vi "Bar graph with LEDs.vi"() -> ()   [LabVIEW 2010]
doc: "This example shows how to make a bar graph by controlling Red Pitaya on board LEDs.\nThe number of LEDs that will be turned ON, corresponds to the value of variable p."
uses:
  RedPitaya.lvlib
panel:
  in  "stop":bool
  in  "Percent":i32 min=0 max=100
  in  "IP address":string="192.168.4.129"
  # "Enter a value between 0 and 100%"
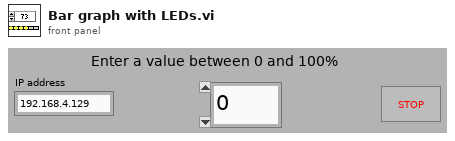
[diagram p1: front panel]
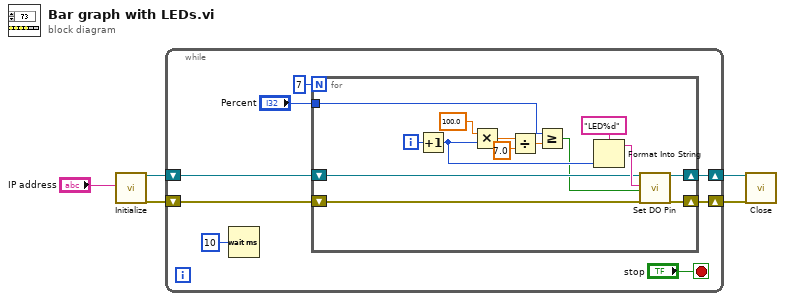
[diagram p0: block diagram]
diagram:
  n1 = call "Initialize.vi"("IP address"="IP address") -> ("RedPitaya connection out"=w2:refnum<k5>, "error out"=w1:errorcluster)  [unwired: 17 in]
  n2 = while {
    shift-right: [w12] -> w4
    shift-left: w2 -> [w10]
    shift-right: [w11] -> w3
    shift-left: w1 -> [w9]
    stop <- "stop" stop-if-true
    n3 = Wait (ms)(milliseconds to wait=u32 10) -> ()  [unwired: 1 out]
    n4 = for {
      N: 7 -> [_]
      tunnel: "Percent" -> [w23]
      shift-right: [w17] -> w12
      shift-left: w10 -> [w18]
      shift-right: [w16] -> w11
      shift-left: w9 -> [w19]
      i -> [w21]
      n5 = Increment(x=w21) -> (x+1=w15:i32)
      n6 = Multiply(x=100.0, y=w15) -> (x*y=w25:dbl)
      n7 = Divide(x=w25, y=7.0) -> (x/y=w27:dbl)
      n8 = Greater Or Equal?(x=w23, y=w27) -> (x >= y?=w14:bool)
      n9 = Format Into String(format string="LED%d", w15) -> (resulting string=w20:string)  [unwired: 2 in, 1 out]
      n10 = call "Set DO Pin.vi"("RedPitaya connection in"=w18, "Pin name"=w20, "State"=w14, "error in"=w19) -> ("RedPitaya connection out"=w17:refnum<k5>, "error out"=w16:errorcluster)  [unwired: 14 in]
    }
  }
  n11 = call "Close.vi"("RedPitaya connection in"=w4, "error in"=w3) -> ()  [unwired: 17 in, 1 out]
